vi "test.vi"() -> ()   [LabVIEW 2010]
uses:
  XComponentSpecification/XComponentSpecification.xctl
  XUserDropdown/XUserDropdown/XUserDropdown.xctl
panel:
  in  "XUserDropdown":string(xcontrol)
  in  "XComponentSpecification":T1(xcontrol)
  out "configuration":string
  in  "Boolean":bool
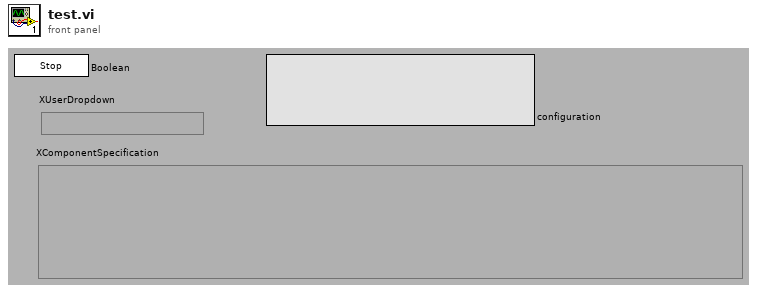
[diagram p1: front panel]
types:
  T1 = cluster{"class path":string, "configuration":string, "label":string, "settings name":string}
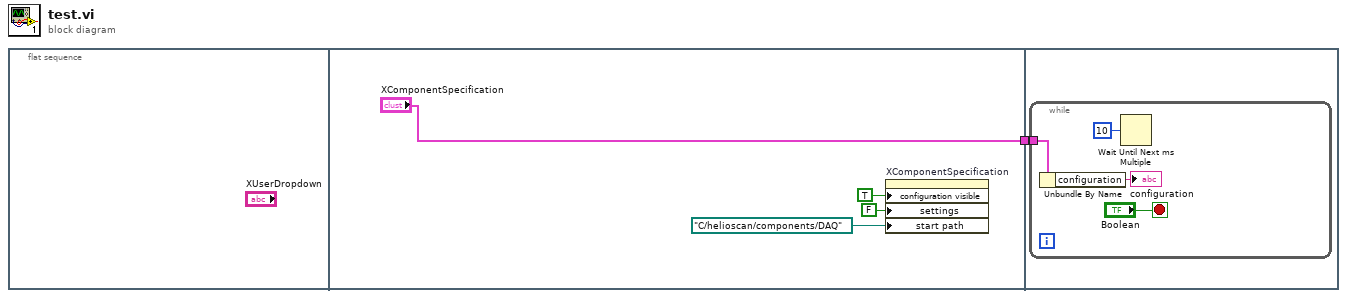
[diagram p0: block diagram]
diagram:
  n1 = flat-sequence {
    tunnel: ["XComponentSpecification"] -> w1
    tunnel: w1 -> [w6]
    frame #0 {
    }
    frame #1 {
      n2 = property on="XComponentSpecification" class="XComponentSpecification (strict"("configuration visible"=TRUE, "settings"=FALSE ("settings visible"), "start path"=path "C:/helioscan/components/DAQ") -> ()  [unwired: 2 in, 2 out]
    }
    frame #2 {
      n3 = while {
        tunnel: w6 -> [w7]
        stop <- "Boolean" stop-if-true
        n4 = Unbundle By Name(w7) -> ("configuration"=→"configuration":string)
        n5 = Wait Until Next ms Multiple(millisecond multiple=u32 10) -> ()  [unwired: 1 out]
      }
    }
  }
